vi "Set Default Value.vi"(9 "Default C++ Value":string, 10 "Control Ref":refnum<vi>, 11 "Enum Writer in":refnum<class "Enum Writer.lvclass">) -> (1 "LabVIEW Default String":string, 2 "Control Ref Dup":refnum<vi>, 3 "Enum Writer out":refnum<class "Enum Writer.lvclass">)   [LabVIEW 2014, in "Enum Writer.lvclass"]
doc: "Copyright (c) 2021 Sze Howe Koh\n\nThis Source Code Form is subject to the terms of the Mozilla Public License, v. 2.0. If a copy of the MPL was not distributed with this file, You can obtain one at http://mozilla.org/MPL/2.0/."
uses:
  Enum Writer.lvclass
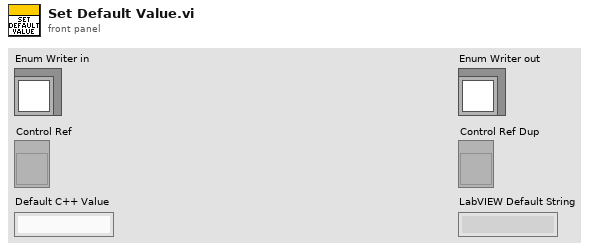
[diagram p1: front panel]
types:
  T1 = typedef "LVStringsAndValuesArrayTypeDef.ctl" = cluster{"String":string, "Value":ext}[]
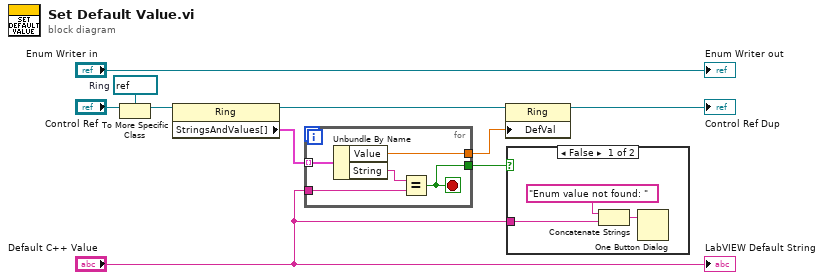
[diagram p0: block diagram]
diagram:
  w7 = refnum<vi> refnum  # Ring
  n1 = To More Specific Class(target class=w7, reference="Control Ref") -> (specific class reference=w6:refnum<vi>)  [unwired: 1 in, 1 out]
  n2 = property class="Ring"(reference=w6) -> (reference out=w5:refnum<vi>, "StringsAndValues[]"=w4:T1)  [unwired: 1 in, 1 out]
  n3 = for {
    tunnel: w4 -> [w15] mode=indexing
    tunnel: "Default C++ Value" -> [w14]
    tunnel: [w12] -> w2
    tunnel: [w11] -> w3
    stop <- w12 stop-if-true
    n4 = Unbundle By Name(w15) -> ("Value"=w11:ext, "String"=w13:string)
    n5 = Equal?(x=w13, y=w14) -> (x = y?=w12:bool)
  }
  n6 = property class="Ring"(reference=w5, "DefVal"=w3) -> (reference out=→"Control Ref Dup":refnum<vi>)  [unwired: 1 in, 1 out]
  n7 = case shown="False" w2 {
    tunnel: "Default C++ Value" -> [w18 _]
    frame False {
      n8 = Concatenate Strings("Enum value not found: " ("string"), w18) -> (w16:string)
      n9 = One Button Dialog(message=w16) -> ()  [unwired: 1 in, 1 out]
    }
    frame True {
    }
  }
  "Enum Writer out" <- "Enum Writer in"
  "LabVIEW Default String" <- "Default C++ Value"
